vi "PTOTeleOp.vi"(10 "Robot":T1, 11 "Buttons":bool[](array[boolean])) -> ()   [LabVIEW 2015]
uses:
  Robot Type Def.ctl
  Framework/JoystickMappingNamesTypeDef.ctl
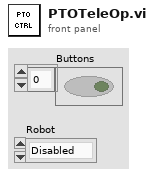
[diagram p1: front panel]
types:
  T1 = typedef "Robot Type Def.ctl" = enum32{"Disabled", "Ghost", "Casper", "Lofty", "Board", "RaceRobot", "Casper 2.0", "Excalibot 2.0"}
  T2 = typedef "JoystickMappingNamesTypeDef.ctl" = enum16{"Shoot Button", "Retrieve Button", "Arm Control", "High Gear", "Low Gear", "Enable PTO", "Disable PTO", "PortC Control", "PortC Up", "PortC Down", "Lift Control", "Drive VBus", "Override Arm Limits"}
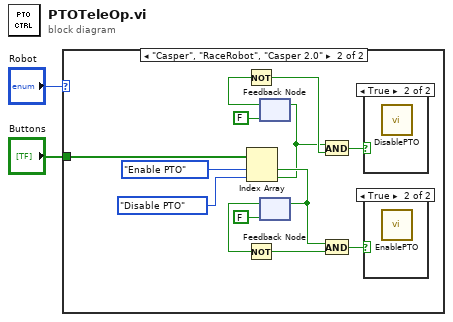
[diagram p0: block diagram]
diagram:
  n1 = case shown="\"Casper\", \"RaceRobot\", \"Casper 2.0\"" "Robot" {
    tunnel: "Buttons" -> [_ w15]
    frame "Disabled", Default {
    }
    frame "Casper", "RaceRobot", "Casper 2.0" {
      n2 = Index Array(array=w15, index #1=JoystickMappingNamesTypeDef."Enable PTO" ("Joystick Button Names"), index #2=JoystickMappingNamesTypeDef."Disable PTO" ("Joystick Button Names")) -> (element #1=w4:bool, element #2=w3:bool)
      n3 = feedback #1(FALSE) -> (w10:bool)
      n4 = Not(x=w10) -> (.not. x?=w11:bool)
      n5 = feedback-in #1(w3) -> ()
      n6 = feedback #2(FALSE) -> (w6:bool)
      n7 = Not(x=w6) -> (.not. x?=w7:bool)
      n8 = feedback-in #2(w4) -> ()
      n9 = And(x=w3, y=w11) -> (x .and. y?=w9:bool)
      n10 = And(x=w4, y=w7) -> (x .and. y?=w5:bool)
      n11 = case shown="True" w9 {
        frame False {
        }
        frame True {
          n12 = call "DisablePTO.vi"() -> ()  [unwired: 11 in, 1 out]
        }
      }
      n13 = case shown="True" w5 {
        frame False {
        }
        frame True {
          n14 = call "EnablePTO.vi"() -> ()  [unwired: 11 in, 1 out]
        }
      }
    }
  }
